vi "PXI-Read AI Buffers.vi"(0 "AI Tasks":T1[](array[typedef]), 1 "Samples to skip":i32, 7 "Samples per channel":i32, 11 "error in (no error)":errorcluster, 12 "timeout (sec)":dbl=10.0 format="%0.2f") -> (4 "AI Tasks out":T1[](array[typedef]), 8 "AI Waveforms":dbl[][](array[numeric]), 15 "error out":errorcluster)   [LabVIEW 2020]
uses:
  Type Defs/Task Struct.ctl
  <vilib>/DAQmx/read.llb/DAQmx Read (Analog 1D DBL 1Chan NSamp).vi
  <vilib>/DAQmx/read.llb/DAQmx Read (Analog 2D DBL NChan NSamp).vi
  <vilib>/DAQmx/miscellaneous.llb/DAQmx Fill In Error Info.vi
  PXI Globals.vi
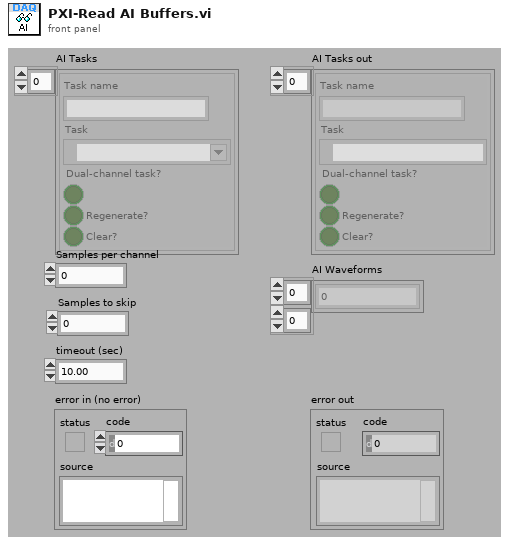
[diagram p1: front panel]
types:
  T1 = typedef "Task Struct.ctl" = cluster{"Task name":string, "Task":refnum<k21>, "Dual-channel task?":bool, "Regenerate?":bool, "Clear?":bool}
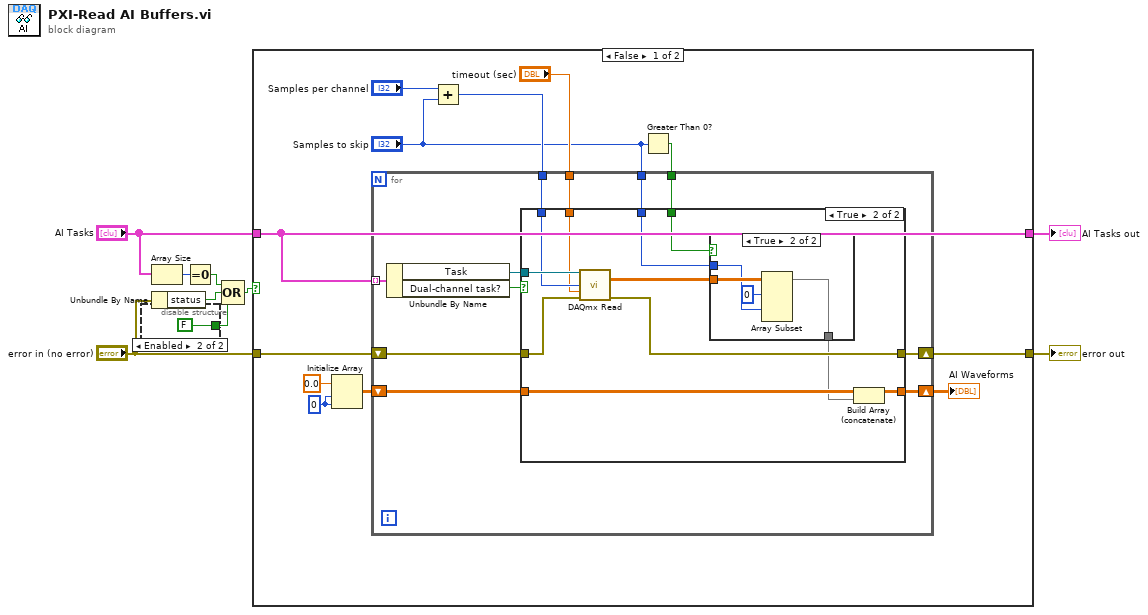
[diagram p0: block diagram]
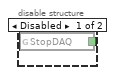
[diagram p2: hidden frame]
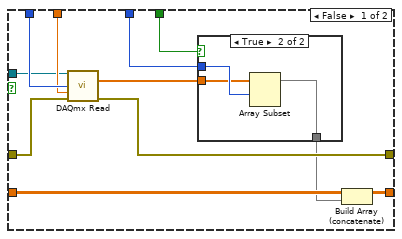
[diagram p3: hidden frame]
diagram:
  n1 = disable-structure shown="Enabled" {
    disable-tunnel: [w10 FALSE ("StopDAQ")] -> w1
    frame Disabled {
      n2 = global read "PXI Globals.vi" "StopDAQ"() -> (w10:bool)
    }
    frame Enabled {
    }
  }
  n3 = Array Size(array="AI Tasks") -> (size(s)=w8:i32)
  n4 = Unbundle By Name("error in (no error)") -> ("status"=w7:bool)
  n5 = Equal To 0?(x=w8) -> (x = 0?=w6:bool)
  n6 = Compound Arithmetic op=OR(w6, w7, w1) -> (w3:bool)
  n7 = case shown="False" w3 {
    tunnel: "error in (no error)" -> [w23 w67]
    tunnel: [w22 w67] -> w9
    tunnel: "AI Tasks" -> [w14 w66]
    tunnel: [w14 w66] -> w2
    frame False {
      w20 = 0 ("dimension size")
      n8 = Initialize Array(0.0 ("element"), w20, w20) -> (w19:dbl[][])
      n9 = Add(x="Samples per channel", y="Samples to skip") -> (x+y=w17:i32)
      n10 = Greater Than 0?(x="Samples to skip") -> (x > 0?=w16:bool)
      n11 = for {
        tunnel: w14 -> [w34] mode=indexing
        shift-right: [w32] -> w22
        shift-left: w23 -> [w33]
        tunnel: w17 -> [w31]
        tunnel: "timeout (sec)" -> [w30]
        shift-right: [w27] -> w12
        shift-left: w19 -> [w28]
        tunnel: w16 -> [w26]
        tunnel: "Samples to skip" -> [w25]
        n12 = Unbundle By Name(w34) -> ("Task"=w24:refnum<k21>, "Dual-channel task?"=w29:bool)
        n13 = case shown="True" w29 {
          tunnel: w33 -> [w45 w60]
          tunnel: [w44 w59] -> w32
          tunnel: w24 -> [w35 w58]
          tunnel: w31 -> [w43 w57]
          tunnel: w30 -> [w42 w56]
          tunnel: w28 -> [w41 w55]
          tunnel: [w40 w54] -> w27
          tunnel: w26 -> [w38 w52]
          tunnel: w25 -> [w37 w51]
          frame False {
            n14 = call-poly <vilib>:"DAQmx Read.vi"("task/channels in"=w35, "number of samples per channel"=w43, "timeout"=w42, "error in"=w45) -> ("data"=w39:dbl[], "error out"=w44:errorcluster)  [unwired: 9 in, 1 out]
            n15 = case shown="True" w38 {
              tunnel: w39 -> [w46 w47]
              tunnel: w37 -> [_ w49]
              tunnel: [w46 w48] -> w36
              frame False {
              }
              frame True {
                n16 = Array Subset(array=w47, index=w49) -> (w48:dbl[])  [unwired: 1 in]
              }
            }
            n17 = Build Array (concatenate)(w41, w36) -> (w40:dbl[][])
          }
          frame True {
            n18 = call-poly <vilib>:"DAQmx Read.vi"("task/channels in"=w58, "number of samples per channel"=w57, "timeout"=w56, "error in"=w60) -> ("data"=w53:dbl[][], "error out"=w59:errorcluster)  [unwired: 9 in, 1 out]
            n19 = case shown="True" w52 {
              tunnel: w53 -> [w61 w65]
              tunnel: w51 -> [_ w63]
              tunnel: [w61 w64] -> w50
              frame False {
              }
              frame True {
                n20 = Array Subset(array=w65, index (row)=0, index (col)=w63) -> (w64:dbl[][])  [unwired: 2 in]
              }
            }
            n21 = Build Array (concatenate)(w55, w50) -> (w54:dbl[][])
          }
        }
      }
      "AI Waveforms" <- w12
    }
    frame True {
    }
  }
  "error out" <- w9
  "AI Tasks out" <- w2
